vi "Current VI's Path (VI or exe).vi"(8 "Error In":errorcluster) -> (0 "Error Out":errorcluster, 3 "VI or executable installation directory":path)   [LabVIEW 2014]
doc: "Current VI's Path (VI or exe).vi\n\n<B>Description:</B>\n\nThe Current VI's Path (VI or exe) VI is a drop-in replacement for the native Current VI's Path function. Just replace the native Current VI's Path function in your application with the Current VI's Path (VI or exe) VI and you'll never have to deal with the frustration caused by bad paths again -- whether you run your code in the development environment or as an executable!\n\nThe Current VI's Path (VI or exe) VI gets the path to the VI that called it and searches that path for \".exe\". If \".exe\" is found in the path, then the Current VI's Path (VI or exe) VI strips the path twice to obtain the executable's installation directory. If \".exe\" is not found, then the Current VI's Path (VI or exe) VI strips the path once to obtain the VI's installation directory.\n\nIn either case, the Current VI's Path (VI or exe) VI returns the VI or executable installation directory and the Full Path to the VI or executable. You can use this information in your application to easily access sub folders of the VI's or executable's installation directory by using the Build Path function to append the sub directory's name to the VI's or executable's installation path returned by the Current VI's Path (VI or exe) VI.\n\n<B>Usage:</B>\n\nUse the Current VI's Path (VI or exe) VI wherever you would use the native Current VI's Path function.\n\n<B>NOTES:</B>\n\nNone.\n\n<B>Inputs:</B>\n\nNone.\n\n<B>Outputs:</B>\n\nFull Path to VI or executable - The full path to the VI or executable.\n\nVI or executable installation directory - The path to the installation directory of the VI or executable.\n\n<B>Developed by:</B>\n\nMark Ridgley\nmark.ridgley@logicpd.com"
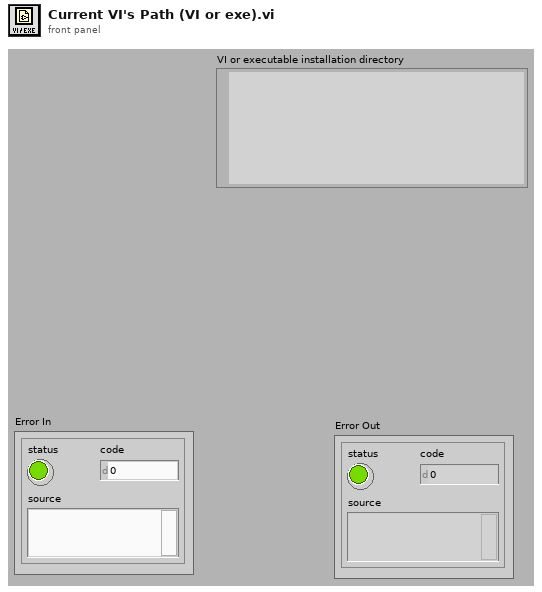
[diagram p1: front panel]
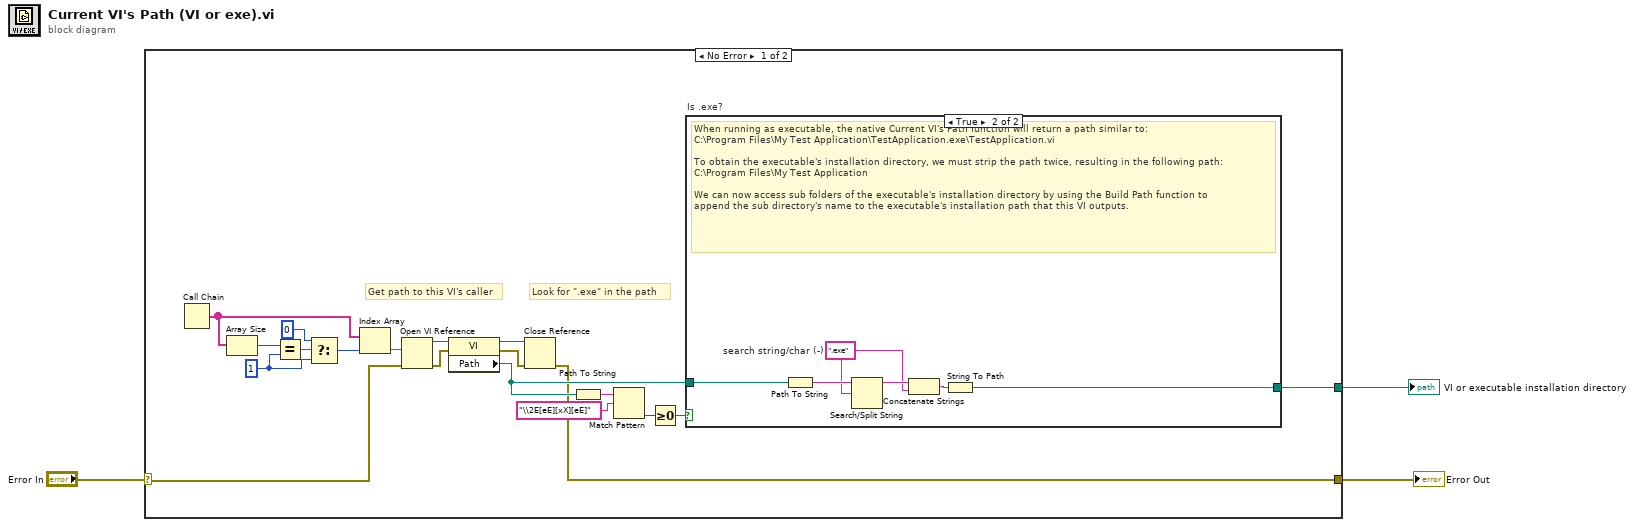
[diagram p0: block diagram]
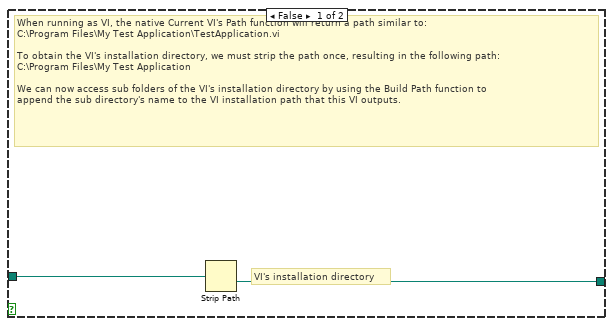
[diagram p2: hidden frame]
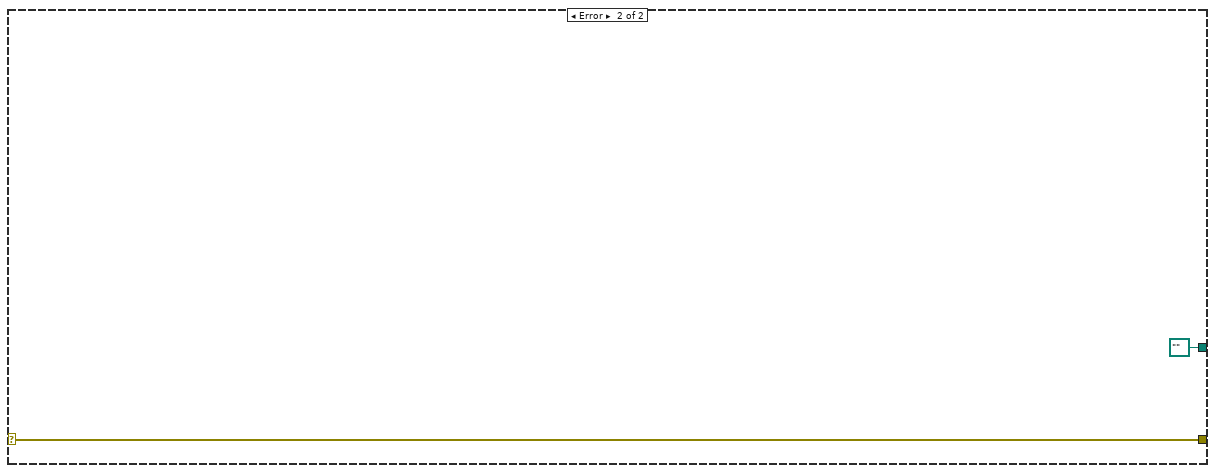
[diagram p3: hidden frame]
diagram:
  n1 = case shown="No Error" "Error In" {
    selector: "Error In" -> [w5 w32]
    tunnel: [w22 path "" ("stripped path")] -> w3
    tunnel: [w4 w32] -> w1
    frame No Error {
      w13 = 1 ("index")
      # "Get path to this VI's caller"
      # "Look for \".exe\" in the path"
      n2 = Call Chain() -> (call chain=w17:string[])
      n3 = Array Size(array=w17) -> (size(s)=w14:i32)
      n4 = Equal?(x=w14, y=w13) -> (x = y?=w16:bool)
      n5 = Select(t=0, s=w16, f=w13) -> (s? t:f=w15:i32)
      n6 = Index Array(array=w17, index=w15) -> (element=w9:string)
      n7 = Open VI Reference(vi path=w9, error in (no error)=w5) -> (vi reference=w10:refnum<vi>, error out=w11:errorcluster)  [unwired: 4 in]
      n8 = property class="VI"(reference=w10, error in=w11) -> (reference out=w6:refnum<vi>, error out=w7:errorcluster, "Path"=w8:path)
      n9 = Close Reference(reference=w6, error in (no error)=w7) -> (error out=w4:errorcluster)
      n10 = Path To String(path=w8) -> (string=w19:string)
      n11 = Match Pattern(string=w19, regular expression="\\2E[eE][xX][eE]") -> (offset past match=w21:i32)  [unwired: 1 in, 3 out]
      n12 = Greater Or Equal To 0?(x=w21) -> (x >= 0?=w20:bool)
      n13 = case "Is .exe?" shown="True" w20 {
        tunnel: w8 -> [w24 w30]
        tunnel: [w23 w25] -> w22
        frame False {
          # "VI's installation directory"
          # "When running as VI, the native Current VI's Path function will return a path similar to:\nC:\\Program Files\\My Test Application\\TestApplication.vi\n\nTo obtain the VI's installation directory, we must strip the path once, resulting in the following path:\nC:\\Program Files\\My Test Application\n\nWe can now access sub folders of the VI's installation directory by using the Build Path function to\nappend the sub directory's name to the VI installation path that this VI outputs."
          n14 = Strip Path(path=w24) -> (stripped path=w23:path)  [unwired: 1 out]
        }
        frame True {
          w27 = ".exe"  # search string/char (-)
          # "When running as executable, the native Current VI's Path function will return a path similar to:\nC:\\Program Files\\My Test Application\\TestApplication.exe\\TestApplication.vi\n\nTo obtain the executable's installation directory, we must strip the path twice, resulting in the following path:\nC:\\Program Files\\My Test Application\n\nWe can now access sub folders of the executable's installation directory by using the Build Path function to\nappend the sub directory's name to the executable's installation path that this VI outputs."
          n15 = Path To String(path=w30) -> (string=w29:string)
          n16 = Search/Split String(string=w29, search string/char (-)=w27) -> (substring before match=w28:string)  [unwired: 1 in, 2 out]
          n17 = Concatenate Strings(w28, w27) -> (w26:string)
          n18 = String To Path(string=w26) -> (path=w25:path)
        }
      }
    }
    frame Error {
    }
  }
  "VI or executable installation directory" <- w3
  "Error Out" <- w1
